vi "AB_820_850_Convert_Path_to_Absolute.vi"(8 "error in (no error)":errorcluster, 9 "relativeType":string, 10 "commonPath":path, 11 "relativePath":path) -> (0 "error out":errorcluster, 3 "absolute path":path)   [LabVIEW 2020]
uses:
  <vilib>/AppBuilder/RW_Project/Compatibility/AB_820_850_Relative_Path_Type.ctl
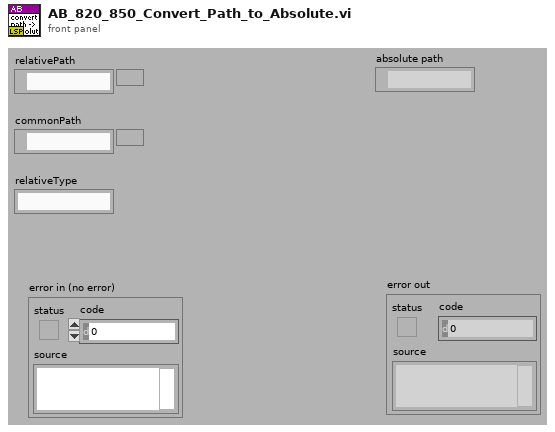
[diagram p1: front panel]
types:
  T1 = typedef "AB_820_850_Relative_Path_Type.ctl" = enum16{"<none>", "relativeToCommon", "relativeToAppDir"}
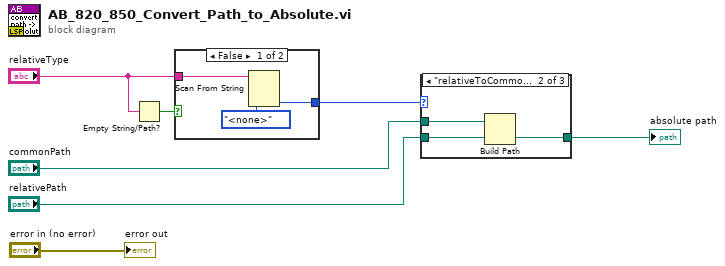
[diagram p0: block diagram]
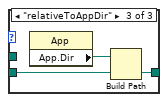
[diagram p3: hidden frame]
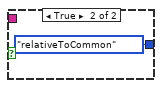
[diagram p4: hidden frame]
diagram:
  n1 = Empty String/Path?(string/path="relativeType") -> (empty?=w2:bool)
  n2 = case shown="False" w2 {
    tunnel: "relativeType" -> [w9 _]
    tunnel: [w8 AB_820_850_Relative_Path_Type."relativeToCommon" ("relativeType")] -> w4
    frame False {
      n3 = Scan From String(input string=w9, default 1=AB_820_850_Relative_Path_Type."<none>" ("relativeType")) -> (output 1=w8:T1)  [unwired: 3 in, 3 out]
    }
    frame True {
    }
  }
  n4 = case shown="\"relativeToCommon\"" w4 {
    tunnel: "relativePath" -> [w12 w15 w18]
    tunnel: [w12 w14 w17] -> w6
    tunnel: "commonPath" -> [_ w13 _]
    frame "<none>" {
      # "absolute path"
    }
    frame "relativeToCommon" {
      n5 = Build Path(base path=w13, name or relative path=w15) -> (appended path=w14:path)
    }
    frame "relativeToAppDir" {
      n6 = property class="App"() -> ("App.Dir"=w16:path)  [unwired: 2 in, 2 out]
      n7 = Build Path(base path=w16, name or relative path=w18) -> (appended path=w17:path)
    }
  }
  "absolute path" <- w6
  "error out" <- "error in (no error)"
